vi "temp.vi"() -> ()   [LabVIEW 2020]
panel:
  out "Pattern":u32[](array[numeric])
  in  "List":i32[][](array[numeric])
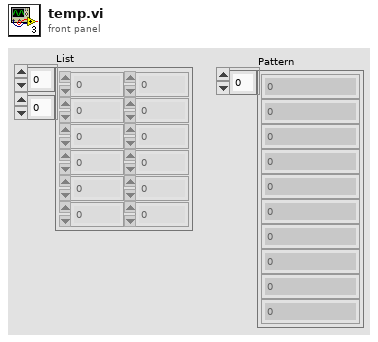
[diagram p1: front panel]
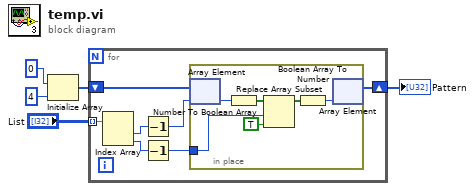
[diagram p0: block diagram]
diagram:
  n1 = Initialize Array(u32 0, 4 ("dimension size")) -> (w2:u32[])
  n2 = for {
    tunnel: "List" -> [w12] mode=indexing
    shift-right: [w10] -> w1
    shift-left: w2 -> [w11]
    n3 = Index Array(array=w12) -> (element #1=w8:i32, element #2=w9:i32)  [unwired: 2 in]
    n4 = Decrement(x=w8) -> (x-1=w7:i32)
    n5 = Decrement(x=w9) -> (x-1=w6:i32)
    n6 = in-place {
      in-place-border: w6 -> [w13]
      n7 = in-place-array #1(w11, w7) -> (w18:u32)
      n8 = Number To Boolean Array(number=w18) -> (Boolean array=w16:bool[])
      n9 = Replace Array Subset(array=w16, new element=TRUE, index=w13) -> (w15:bool[])
      n10 = Boolean Array To Number(Boolean array=w15) -> (number=w14:u32)
      n11 = in-place-array #1(w14) -> (w10:u32[])  [unwired: 1 out]
    }
  }
  "Pattern" <- w1
